vi "Exercise2.vi"() -> ()   [LabVIEW 2019]
panel:
  out "Numeric Case Structure\nIndicator":string
  in  "Temperature\nControl":dbl min=0.0 max=100.0 step=5.0
  out "Nested Case Structure\n Indicator":string
  out "Thermometer":dbl(slide) scale=0.0..100.0
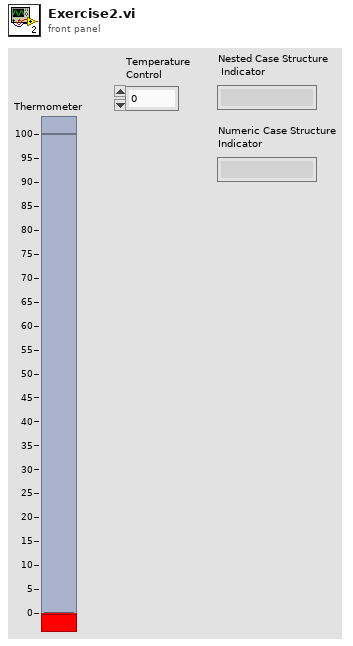
[diagram p1: front panel]
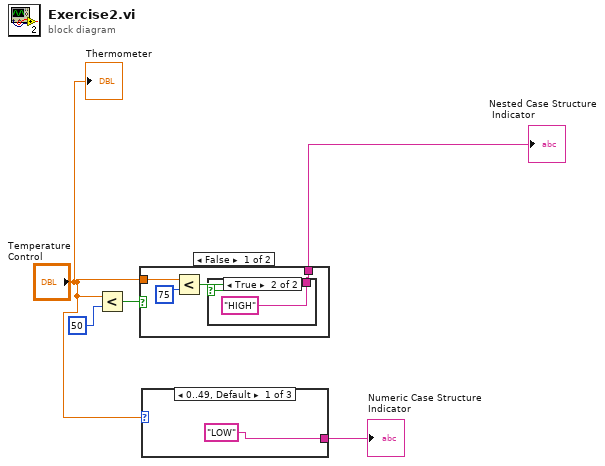
[diagram p0: block diagram]
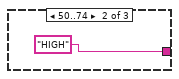
[diagram p2: hidden frame]
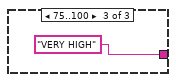
[diagram p3: hidden frame]
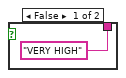
[diagram p4: hidden frame]
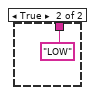
[diagram p5: hidden frame]
diagram:
  n1 = Less?(x="Temperature\nControl", y=50) -> (x < y?=w4:bool)
  n2 = case shown="False" w4 {
    tunnel: [w6 "LOW"] -> w3
    tunnel: "Temperature\nControl" -> [w8 _]
    frame False {
      n3 = Less?(x=w8, y=75) -> (x < y?=w9:bool)
      n4 = case shown="True" w9 {
        tunnel: ["VERY HIGH" "HIGH"] -> w6
        frame False {
        }
        frame True {
        }
      }
    }
    frame True {
    }
  }
  "Nested Case Structure\n Indicator" <- w3
  n5 = case shown="0..49, Default" "Temperature\nControl" {
    tunnel: ["LOW" "HIGH" "VERY HIGH"] -> w1
    frame 0..49, Default {
    }
    frame 50..74 {
    }
    frame 75..100 {
    }
  }
  "Numeric Case Structure\nIndicator" <- w1
  "Thermometer" <- "Temperature\nControl"
